vi "Tektronix Test.vi"() -> ()   [LabVIEW 2020]
uses:
  Tektronix Driver/Tektronix Configuration.ctl
  Tektronix MSO 6/Tektronix MSO 6 Driver.lvclass
  C:/GitHub/NHMFL_Core/Libraries/Instruments/Tektronix/Tektronix Driver/Tektronix Driver.lvclass
panel:
  out "Waveform Graph":waveform(dbl)[](graph)
  in  "Tektronix Configuration":T1={"Channel"=1, "Number of averages"=4096, "Input impedace"=enum."1 M Ohm", "Vertical coupling"=enum."AC"}
  in  "VISA resource name":refnum<visa-resource-name>
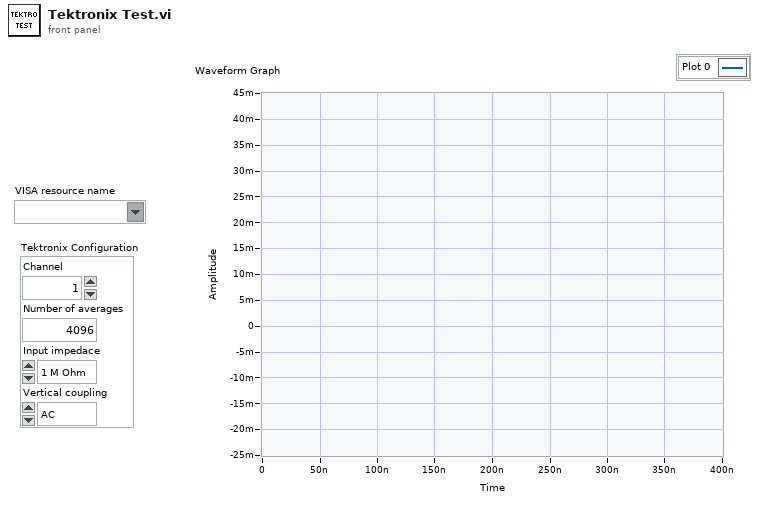
[diagram p1: front panel]
types:
  T1 = typedef "Tektronix Configuration.ctl" = cluster{"Channel":i32, "Number of averages":i32, "Input impedace":enum16{"1 M Ohm", "50 Ohm"}, "Vertical coupling":enum16{"AC", "DC", "Ground"}}
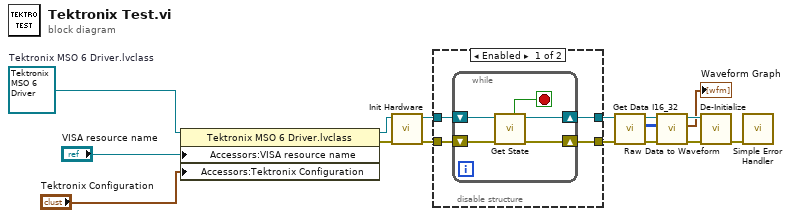
[diagram p0: block diagram]
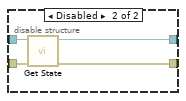
[diagram p2: hidden frame]
diagram:
  w16 = refnum<class "Tektronix MSO 6 Driver.lvclass"> refnum  # Tektronix MSO 6 Driver.lvclass
  n1 = property class="Tektronix MSO 6 Driver.lvclass"(reference=w16, "Accessors:VISA resource name"="VISA resource name", "Accessors:Tektronix Configuration"="Tektronix Configuration") -> (reference out=w15:refnum<class "Tektronix MSO 6 Driver.lvclass">, error out=w13:errorcluster)  [unwired: 1 in]
  n2 = call-dynamic "Init Hardware.vi"("error in (no error)"=w13, "Tektronix MSO 6 Driver in"=w15) -> ("error out"=w11:errorcluster, "Tektronix MSO 6 Driver out"=w10:refnum<class "Tektronix MSO 6 Driver.lvclass">)  [unwired: 8 in]
  n3 = disable-structure shown="Enabled" {
    disable-tunnel: w11 -> [w20 w28]
    disable-tunnel: w10 -> [w19 w26]
    disable-tunnel: [w18 w27] -> w3
    disable-tunnel: [w17 w29] -> w6
    frame Enabled {
      n4 = while {
        shift-right: [w22] -> w18
        shift-left: w19 -> [w24]
        shift-right: [w23] -> w17
        shift-left: w20 -> [w25]
        stop <- w21 stop-if-true
        n5 = call-dynamic "Get State.vi"("error in (no error)"=w25, "Tektronix MSO 6 Driver in"=w24) -> ("error out"=w23:errorcluster, "Tektronix MSO 6 Driver out"=w22:refnum<class "Tektronix MSO 6 Driver.lvclass">, "Finished"=w21:bool)  [unwired: 4 in, 3 out]
      }
    }
    frame Disabled {
      n6 = call-dynamic "Get State.vi"("error in (no error)"=w28, "Tektronix MSO 6 Driver in"=w26) -> ("error out"=w29:errorcluster, "Tektronix MSO 6 Driver out"=w27:refnum<class "Tektronix MSO 6 Driver.lvclass">)  [unwired: 4 in, 4 out]
    }
  }
  n7 = call-dynamic "Get Data I16_32.vi"("error in (no error)"=w6, "Tektronix MSO 6 Driver in"=w3) -> ("error out"=w5:errorcluster, "I16 data out"=w4:i16[][], "Tektronix MSO 6 Driver out"=w2:refnum<class "Tektronix MSO 6 Driver.lvclass">)  [unwired: 4 in, 3 out]
  n8 = call-dynamic "Raw Data to Waveform.vi"("error in (no error)"=w5, "I16 data"=w4, "Pulse Driver in"=w2) -> ("error out"=w7:errorcluster, "Array"=→"Waveform Graph":waveform(dbl)[], "Pulse Driver out"=w8:refnum<class "Tektronix MSO 6 Driver.lvclass">)  [unwired: 6 in]
  n9 = call-dynamic "De-Initialize.vi"("error in (no error)"=w7, "Tektronix MSO 6 Driver in"=w8) -> ("error out"=w9:errorcluster)  [unwired: 8 in, 1 out]
  n10 = call <vilib>:"Simple Error Handler.vi"("error in (no error)"=w9) -> ()  [unwired: 4 in, 5 out]
